vi "KE622x -- Get Math Result.vi"(0 "Resource In":refnum<visa-resource-name>, 1 "Check For SCPI Errors? (T)":bool=TRUE, 7 "Result Type":T1, 11 "error in (no error)":errorcluster) -> (4 "Resource Out (dupl)":refnum<visa-resource-name>, 8 "Math Results":T2 {"Y Value" format="%.6e"; "X Value" format="%.6e"}, 15 "error out":errorcluster)   [LabVIEW 2019, in "Keithley 622x.lvlib"]
doc: "Returns the mathematically modified value of either the last reading ('Latest') or a new reading ('Fresh'). Note that the use of this VI assumes that a Model 2182/2182A nano-voltmeter is connected via the RS232 link (user is performing a Delta, Pulsed Delta, or Differential Conductance measurement), since the 622x doesn't make measurements on its own. If the user selects 'Latest' and a new measurement is not available yet, the last reading will be returned. Selecting 'Fresh' guarantees that a single reading is returned only once -- if a reading is not available, error -230 is returned (Data corrupt or stale)."
uses:
  Keithley 622x.lvlib
  Typedefs/KE622x -- Math Results.ctl
  Typedefs/KE622x -- Math Result Type.ctl
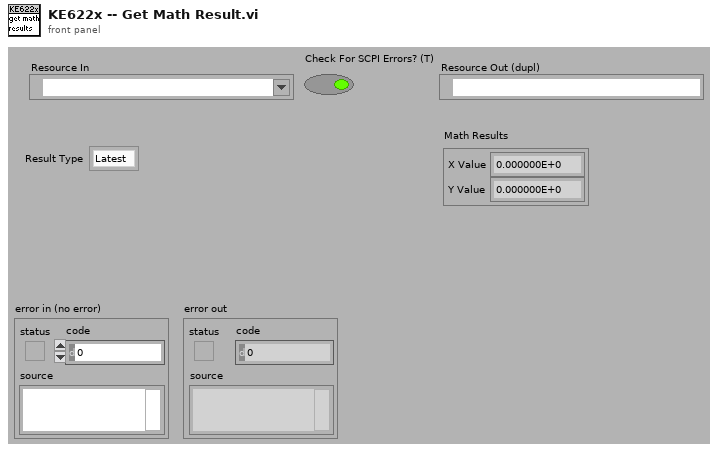
[diagram p1: front panel]
types:
  T1 = typedef "Keithley 622x.lvlib/KE622x -- Math Result Type.ctl" = enum16{"Latest", "Fresh"}
  T2 = typedef "Keithley 622x.lvlib/KE622x -- Math Results.ctl" = cluster{"X Value":dbl, "Y Value":dbl}
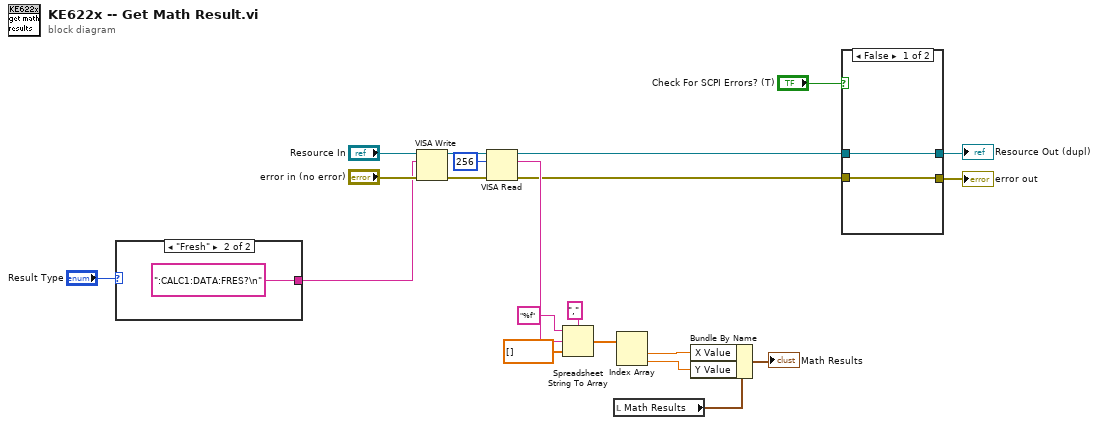
[diagram p0: block diagram]
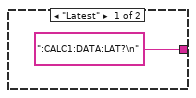
[diagram p2: hidden frame]
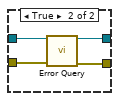
[diagram p3: hidden frame]
diagram:
  n1 = case shown="\"Fresh\"" "Result Type" {
    tunnel: [":CALC1:DATA:LAT?\n" ":CALC1:DATA:FRES?\n"] -> w11
    frame "Latest" {
    }
    frame "Fresh" {
    }
  }
  n2 = VISA Write(VISA resource name="Resource In", write buffer=w11, error in (no error)="error in (no error)") -> (VISA resource name out=w16:refnum<visa-resource-name>, error out=w15:errorcluster)  [unwired: 1 out]
  n3 = VISA Read(VISA resource name=w16, byte count=u32 256, error in (no error)=w15) -> (VISA resource name out=w13:refnum<visa-resource-name>, read buffer=w7:string, error out=w6:errorcluster)  [unwired: 1 out]
  n4 = Spreadsheet String To Array(delimiter (Tab)=",", format string="%f", spreadsheet string=w7, array type (2D Dbl)=dbl[] []) -> (array=w5:dbl[])
  n5 = local read "Math Results"() -> (w4:T2)
  n6 = Index Array(array=w5) -> (element #1=w3:dbl, element #2=w2:dbl)  [unwired: 2 in]
  n7 = Bundle By Name(cluster=w4, "X Value"=w3, "Y Value"=w2) -> (→"Math Results":T2)
  n8 = case shown="False" "Check For SCPI Errors? (T)" {
    tunnel: w13 -> [w25 w29]
    tunnel: w6 -> [w24 w28]
    tunnel: [w24 w27] -> w17
    tunnel: [w25 w26] -> w18
    frame False {
    }
    frame True {
      n9 = call "Error Query.vi"("VISA Resource In"=w29, "error in (no error)"=w28) -> ("VISA Resource Out (dupl)"=w26:refnum<visa-resource-name>, "error out"=w27:errorcluster)  [unwired: 10 in, 2 out]
    }
  }
  "Resource Out (dupl)" <- w18
  "error out" <- w17
